vi "Create DID.vi"(8 "error in (no error)":errorcluster, 10 "DIDPID":T2 {"Signals"."Byte Order" items=["Little Endian", "Big Endian"]; "Signals"."Data Type" items=["Signed", "Unsigned", "IEEE Float"]}, 11 "Section Ptr":T1 format="%.0x") -> (0 "error out":errorcluster, 3 "Parent Ref out":T1 format="%.0x")   [LabVIEW 2015, in "Diagnostics Addon Shared.lvlib"]
uses:
  Diagnostics Addon Shared.lvlib
  DIDPID Parameters.ctl
  DIDPID Signal Parameters.ctl
  <vilib>/NI Veristand/Custom Device API/Custom Device Item Ref.ctl
  GUID Lookup.vi
  <vilib>/NI Veristand/Custom Device API/Custom Device API.lvlib
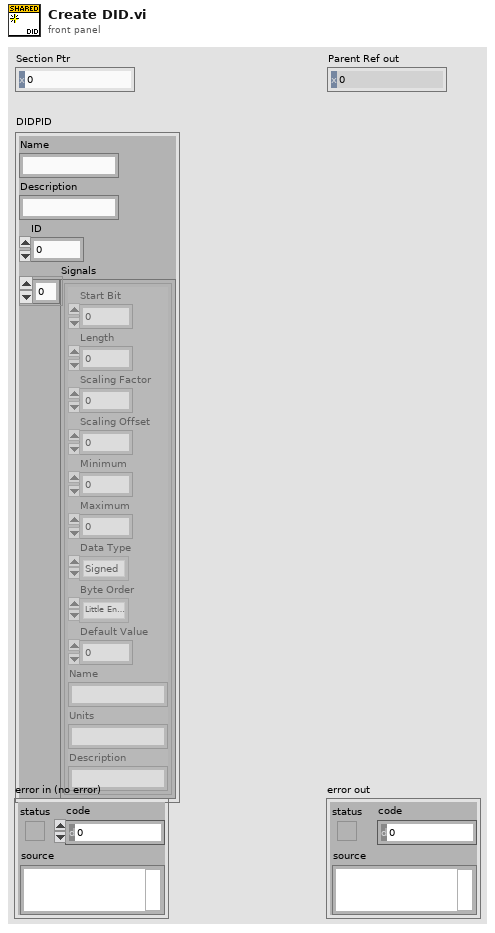
[diagram p1: front panel]
types:
  T1 = typedef "Custom Device API.lvlib/Custom Device Item Ref.ctl" = u64
  T2 = typedef "Diagnostics Addon Shared.lvlib/DIDPID Parameters.ctl" = cluster{"Name":string, "Description":string, "ID":u16, "Signals":T3[]}
  T3 = typedef "Diagnostics Addon Shared.lvlib/DIDPID Signal Parameters.ctl" = cluster{"Start Bit":u8, "Length":u8, "Scaling Factor":dbl, "Scaling Offset":dbl, "Minimum":dbl, "Maximum":dbl, "Data Type":u32, "Byte Order":u32, "Default Value":dbl, "Name":string, "Units":string, "Description":string}
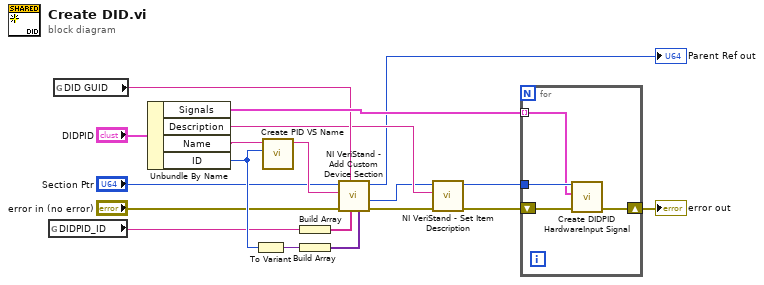
[diagram p0: block diagram]
diagram:
  n1 = global read "GUID Lookup.vi" "DIDPID_ID"() -> (w12:string)
  n2 = global read "GUID Lookup.vi" "DID GUID"() -> (w9:string)
  n3 = Unbundle By Name("DIDPID") -> ("Signals"=w16:T3[], "Description"=w8:string, "Name"=w17:string, "ID"=w18:u16)
  n4 = To Variant(anything=w18) -> (Variant=w13:variant)
  n5 = call "Create PID VS Name.vi"("PID Number"=w18, "PID Name"=w17) -> ("VS Name"=w19:string)  [unwired: 9 in]
  n6 = Build Array(w12) -> (w11:string[])
  n7 = Build Array(w13) -> (w14:variant[])
  n8 = call <vilib>:"NI VeriStand - Add Custom Device Section.vi"("Property Values"=w14, "Property names"=w11, "GUID (Default Section)"=w9, "error in (no error)"="error in (no error)", "Section Name"=w19, "Parent Ref in"="Section Ptr") -> ("error out"=w7:errorcluster, "Section Ptr"=w6:T1, "Parent Ref out"=→"Parent Ref out":T1)  [unwired: 2 in, 1 out]
  n9 = call <vilib>:"NI VeriStand - Set Item Description.vi"("error in (no error)"=w7, "Description"=w8, "Item Ref in"=w6) -> ("error out"=w4:errorcluster, "Item Ref out"=w5:T1)  [unwired: 6 in, 1 out]
  n10 = for {
    shift-right: [w22] -> w15
    shift-left: w4 -> [w23]
    tunnel: w16 -> [w20] mode=indexing
    tunnel: w5 -> [w21]
    n11 = call "Create DIDPID HardwareInput Signal.vi"("error in (no error)"=w23, "Signal Parameters"=w20, "Section Ptr"=w21) -> ("error out"=w22:errorcluster)  [unwired: 7 in, 1 out]
  }
  "error out" <- w15
